vi "master_GUI.vi"() -> ()   [LabVIEW 2018]
panel:
  in  "power":bool
  in  "sec":dbl
  in  "min":dbl
  in  "hour":dbl
  in  "stopwatch":bool
  in  "timer":bool
  in  "setTime":dbl
  in  "time":dbl
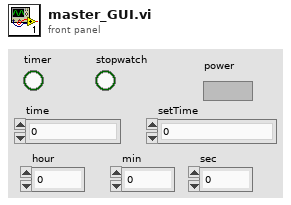
[diagram p1: front panel]
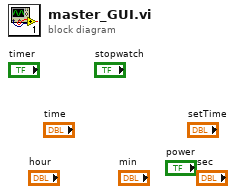
[diagram p0: block diagram]
diagram:
